vi "Configure TIS Mode.vi"(8 "error in":errorcluster, 10 "TIS Mode":T2 items=["TIS Mode (CH0 Only)"=1, "TIS Mode (CH1 Only)"=2, "Dual TIS Mode (CH0 and CH1)"=3], 11 "Ref in":T1) -> (0 "error out":errorcluster, 1 "range (Vpp)":dbl=1.3, 2 "TIS Configured?":bool, 3 "Ref out":T1)   [LabVIEW 2015, in "7976R_v1.lvclass"]
doc: "This VI configures the Time Interleaved Sampling (TIS) for the NI 5772. For execution steps, refer to the comments on the block diagram."
uses:
  <userlib>/SE-APP-Receiver/NI5772/7976R_v1/7976R_v1.lvclass
  <userlib>/SE-APP-Receiver/NI5772/7976R_v1/Private/TIS Mode_v1.ctl
  <userlib>/SE-APP-Receiver/NI5772/7976R_v1/Private/FPGA VI Reference_DDC_v1.8.ctl
  <vilib>/Utility/error.llb/Error Cluster From Error Code.vi
  <vilib>/rvi/errors/niLvFpgaAdjustHostInterfaceError.vi
  <vilib>/rvi/interface/nirviReadWriteControl/nirviReadWriteControl.xnode
  <vilib>/rvi/interface/Simulation/niFpgaSimulationCallBeginRW.vi
  NiFpgaLv.dll
panel:
  # "This VI configures the Time Interleaved Sampling (TIS) for the NI 5771. For execution steps, refer to the comments on the block diagram."
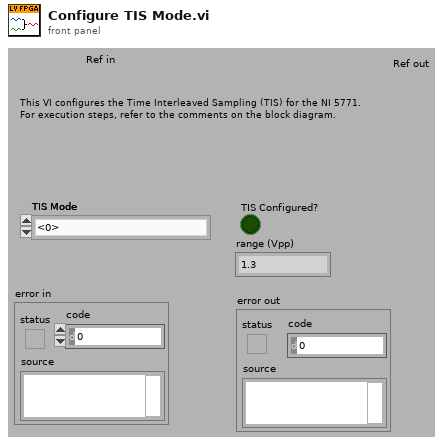
[diagram p1: front panel]
types:
  T1 = typedef "7976R_v1.lvclass/FPGA VI Reference_DDC_v1.8.ctl" = refnum<k20>
  T2 = typedef "7976R_v1.lvclass/TIS Mode_v1.ctl" = u16
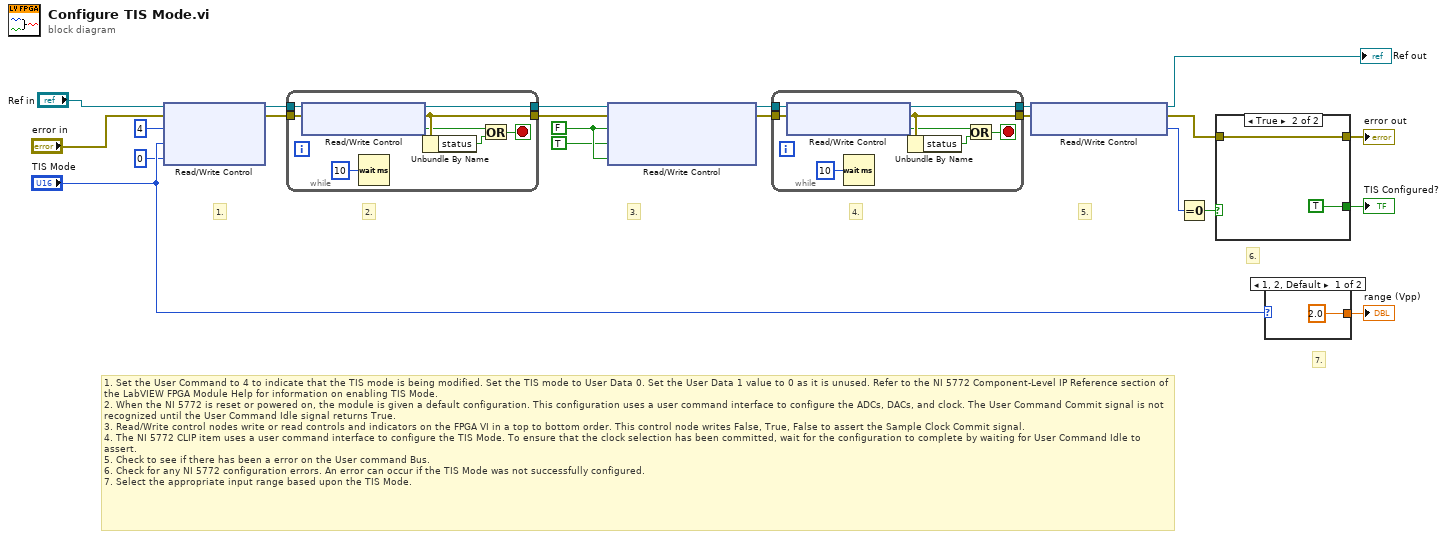
[diagram p0: block diagram]
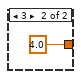
[diagram p2: hidden frame]
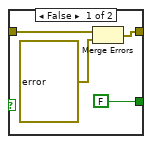
[diagram p3: hidden frame]
diagram:
  w17 = FALSE ("Sample Clock Commit")
  # "7."
  # "5."
  # "1. Set the User Command to 4 to indicate that the TIS mode is being modified. Set the TIS mode to User Data 0. Set the User Data 1 value to 0 as it is unused. Refer to the NI 5772 Component-Level IP Reference section of the LabVIEW FPGA Module Help for information on enabling TIS Mode.\n2. When the NI 5772 is reset or powered on, the module is given a default configuration. This configuration uses a user command interface to configure the ADCs, DACs, and clock. The User Command Commit signal is not recognized until the User Command Idle signal returns True.\n3. Read/Write control nodes write or read controls and indicators on the FPGA VI in a top to bottom order. This control node writes False, True, False to assert the Sample Clock Commit signal.\n4. The NI 5772 CLIP item uses a user command interface to configure the TIS Mode. To ensure that the clock selection has been committed, wait for the configuration to complete by waiting for User Command Idle to assert.\n5. Check to see if there has been a error on the User command Bus.\n6. Check for any NI 5772 configuration errors. An error can occur if the TIS Mode was not successfully configured.\n7. Select the appropriate input range based upon the TIS Mode."
  # "6."
  # "4."
  # "3."
  # "2."
  # "1."
  n1 = xnode "Read/Write Control"("FPGA VI Reference In"="Ref in", "error in"="error in", "User Command"=u8 4, "User Data 0"="TIS Mode", "User Data 1"=u8 0) -> ("FPGA VI Reference Out"=w21:T1, "error out"=w20:errorcluster)
  n2 = while {
    tunnel: w21 -> [w26]
    tunnel: w20 -> [w27]
    tunnel: [w24] -> w18
    tunnel: [w25] -> w19
    stop <- w28 stop-if-true
    n3 = xnode "Read/Write Control"("FPGA VI Reference In"=w26, "error in"=w27) -> ("FPGA VI Reference Out"=w25:T1, "error out"=w24:errorcluster, "User Command Idle"=w23:bool)
    n4 = Wait (ms)(milliseconds to wait=u32 10) -> ()  [unwired: 1 out]
    n5 = Unbundle By Name(w24) -> ("status"=w29:bool)
    n6 = Or(x=w23, y=w29) -> (x .or. y?=w28:bool)
  }
  n7 = xnode "Read/Write Control"("FPGA VI Reference In"=w19, "error in"=w18, "User Command Commit"=w17, "User Command Commit"=TRUE ("Sample Clock Commit"), "User Command Commit"=w17) -> ("FPGA VI Reference Out"=w14:T1, "error out"=w13:errorcluster)
  n8 = while {
    tunnel: w14 -> [w34]
    tunnel: w13 -> [w35]
    tunnel: [w32] -> w12
    tunnel: [w33] -> w11
    stop <- w36 stop-if-true
    n9 = xnode "Read/Write Control"("FPGA VI Reference In"=w34, "error in"=w35) -> ("FPGA VI Reference Out"=w33:T1, "error out"=w32:errorcluster, "User Command Idle"=w31:bool)
    n10 = Wait (ms)(milliseconds to wait=u32 10) -> ()  [unwired: 1 out]
    n11 = Unbundle By Name(w32) -> ("status"=w37:bool)
    n12 = Or(x=w31, y=w37) -> (x .or. y?=w36:bool)
  }
  n13 = xnode "Read/Write Control"("FPGA VI Reference In"=w11, "error in"=w12) -> ("FPGA VI Reference Out"=→"Ref out":T1, "error out"=w9:errorcluster, "User Command Status"=w7:u8)
  n14 = Equal To 0?(x=w7) -> (x = 0?=w6:bool)
  n15 = case shown="True" w6 {
    tunnel: [w42 w44] -> w15
    tunnel: w9 -> [w41 w44]
    tunnel: [FALSE ("Configured?") TRUE ("Configured?")] -> w8
    frame False {
      n16 = Merge Errors(w41, errorcluster {"status"=TRUE, "code"=-8998, "source"="IO Module clock not configured correctly. Please ensure that the desired clock meets the required specifications."} ("error in")) -> (w42:errorcluster)
    }
    frame True {
    }
  }
  "error out" <- w15
  "TIS Configured?" <- w8
  n17 = case shown="1, 2, Default" "TIS Mode" {
    tunnel: [2.0 4.0] -> w5
    frame 1, 2, Default {
    }
    frame 3 {
    }
  }
  "range (Vpp)" <- w5
